vi "writeRTTimestampSV.vi"(8 "error in (no error)":errorcluster, 10 "RTTimestamp":dbl, 11 "ComponentData in":refnum<class "ComponentData.lvclass">) -> (0 "error out":errorcluster, 3 "ComponentData out":refnum<class "ComponentData.lvclass">)   [LabVIEW 2013, in "ComponentData.lvlib" / "ComponentData.lvclass"]
uses:
  <userlib>/Common/Component/common_application/RT/ComponentData/ComponentData/ComponentData.lvclass
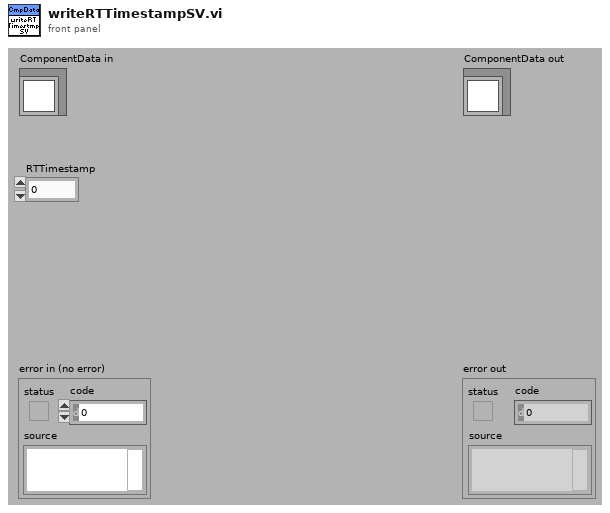
[diagram p1: front panel]
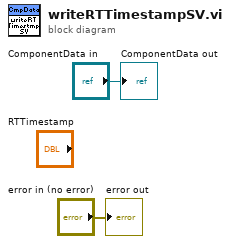
[diagram p0: block diagram]
diagram:
  "error out" <- "error in (no error)"
  "ComponentData out" <- "ComponentData in"
